vi "HH_FileToImage_2.vi"(0 "Data In":u32[](array[numeric]), 1 "Reset":bool, 2 "Image Data In":u16[][][](array[numeric]), 5 "Data Count":i32, 7 "Trigger Times":u64[](array[numeric]), 9 "Trigger":dbl[](array[numeric])) -> (3 "Image Data Out":u16[][][](array[numeric]), 6 "Total Photon Count":u64[](array[numeric]), 13 "Total Oveflow Count":u64, 14 "Num Records Total":i64)   [LabVIEW 2009]
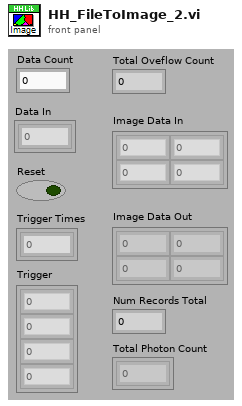
[diagram p1: front panel]
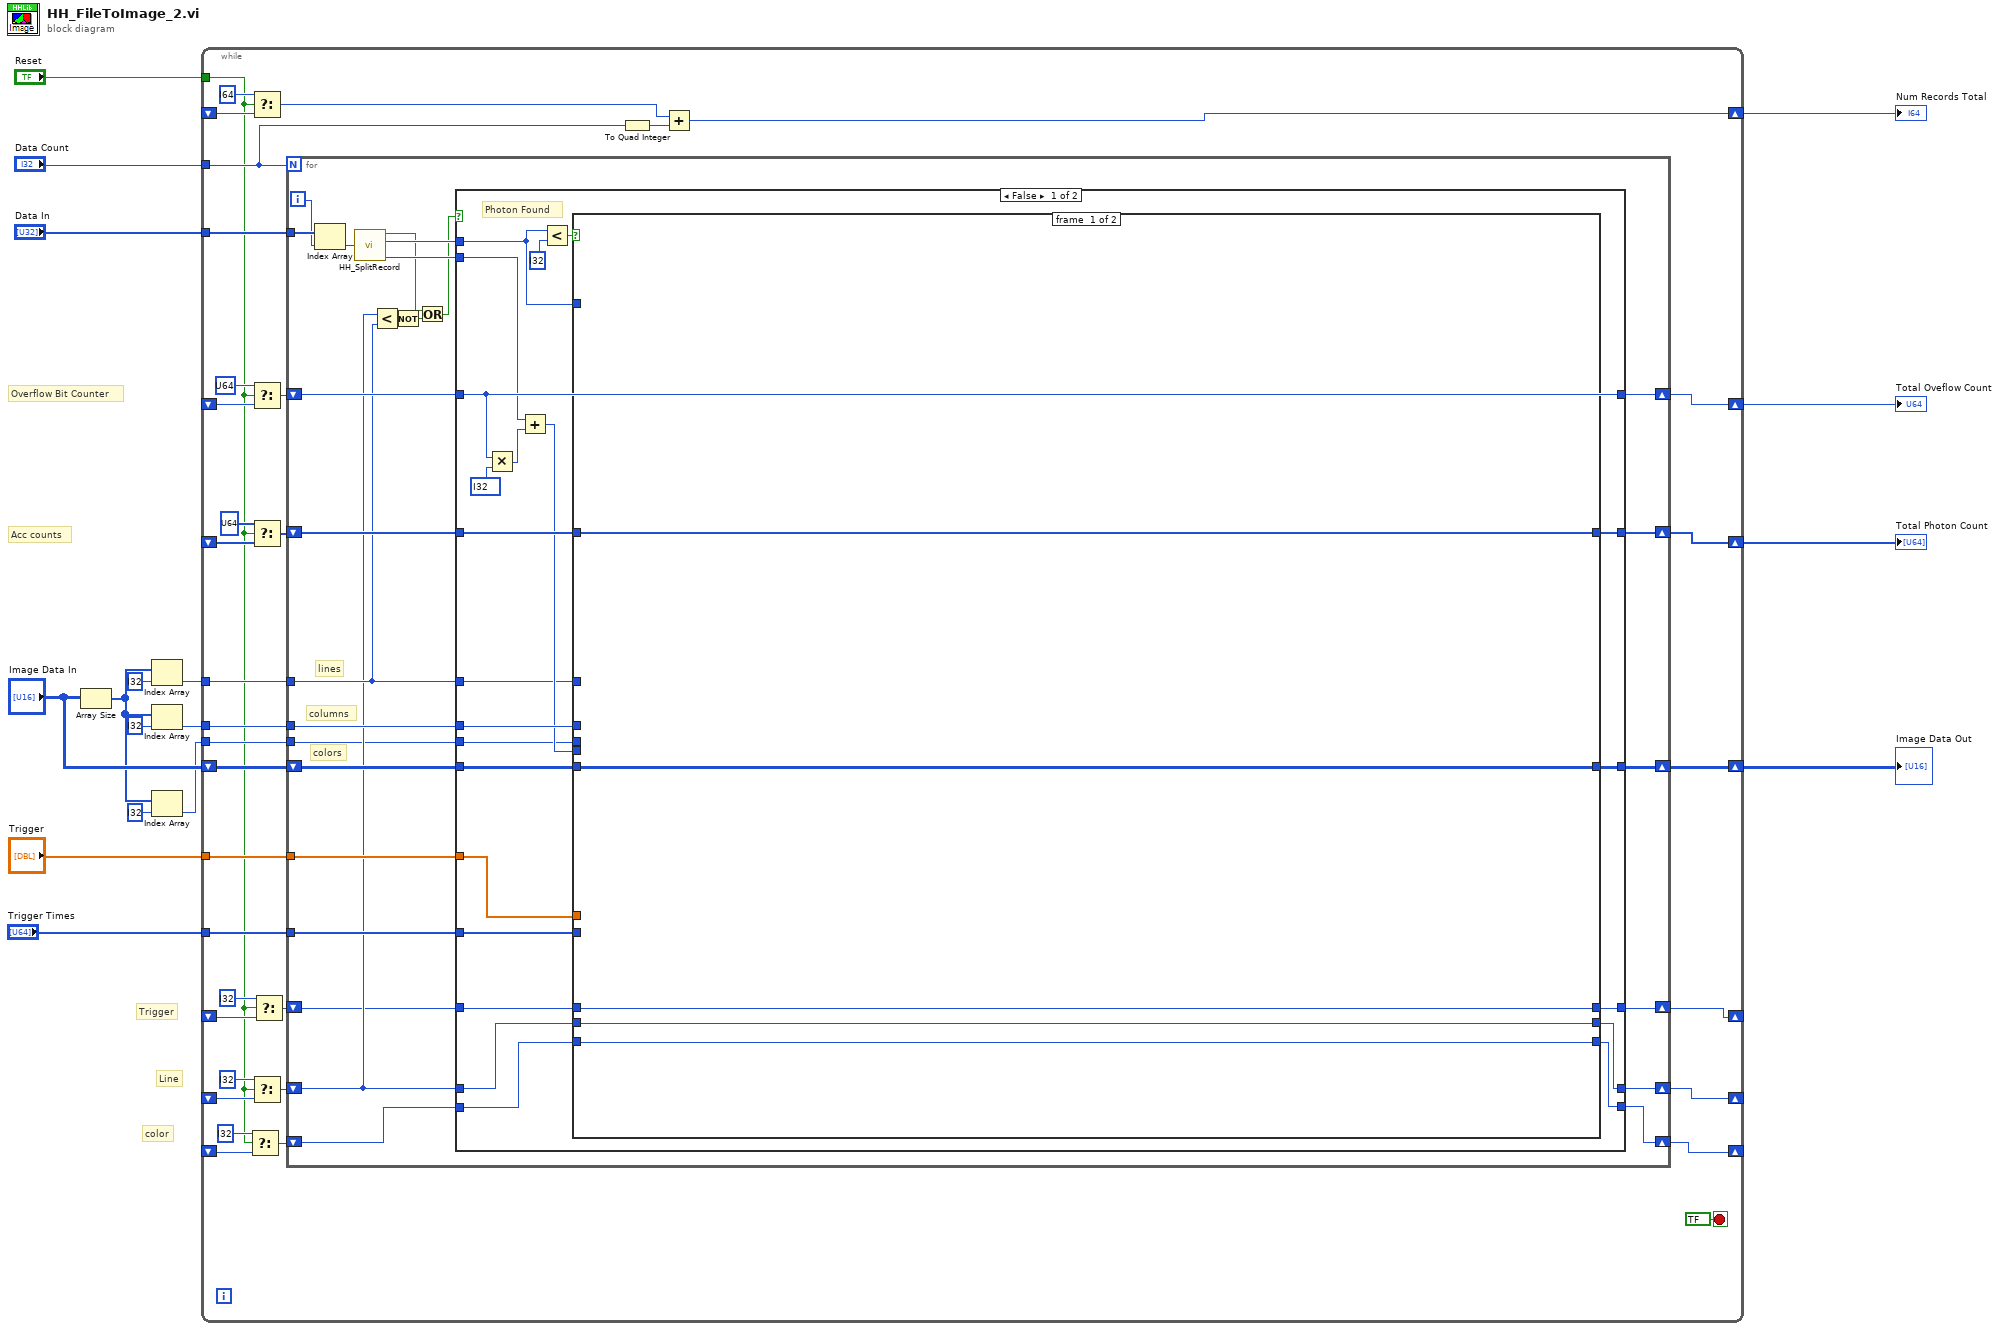
[diagram p0: block diagram]
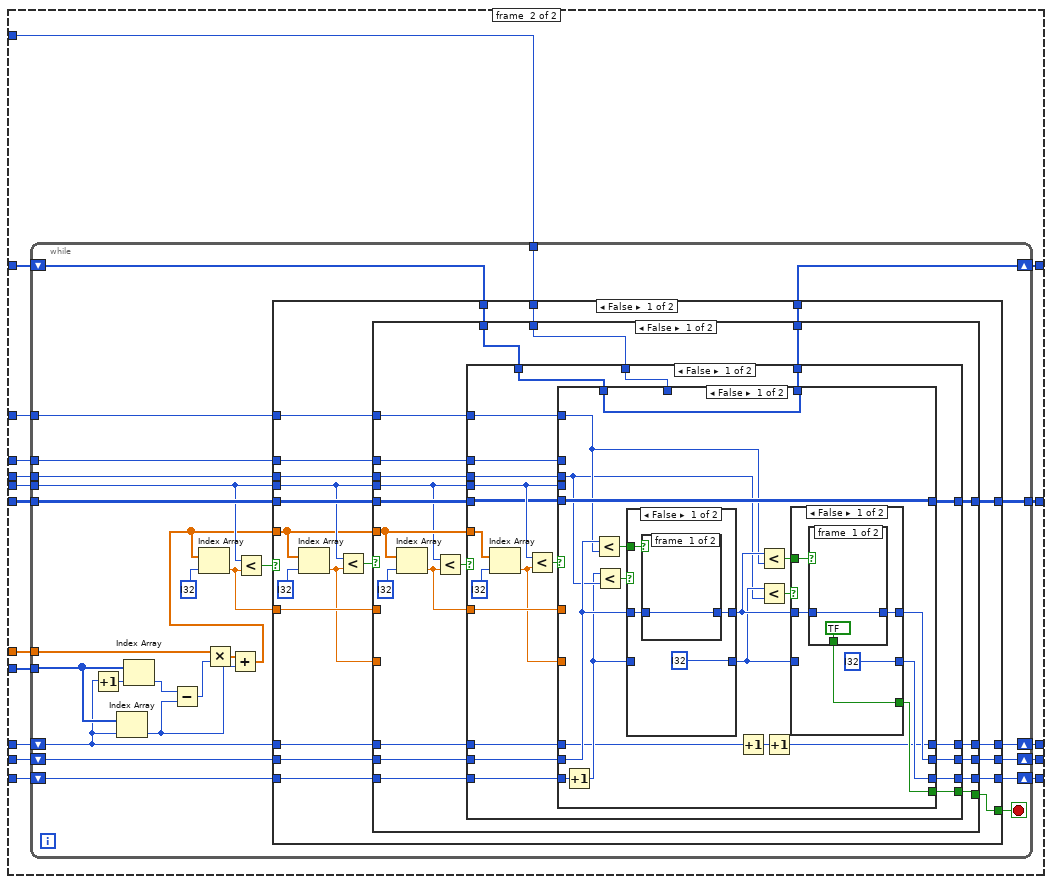
[diagram p2: hidden frame]
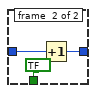
[diagram p3: hidden frame]
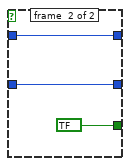
[diagram p4: hidden frame]
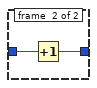
[diagram p5: hidden frame]
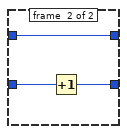
[diagram p6: hidden frame]
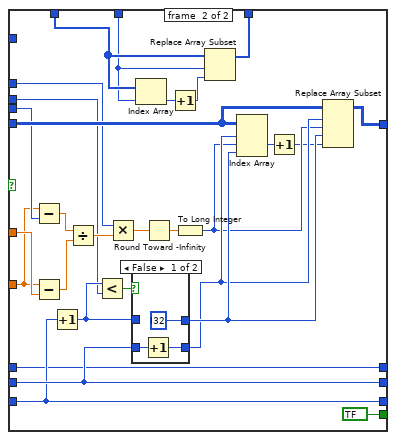
[diagram p7: hidden frame]
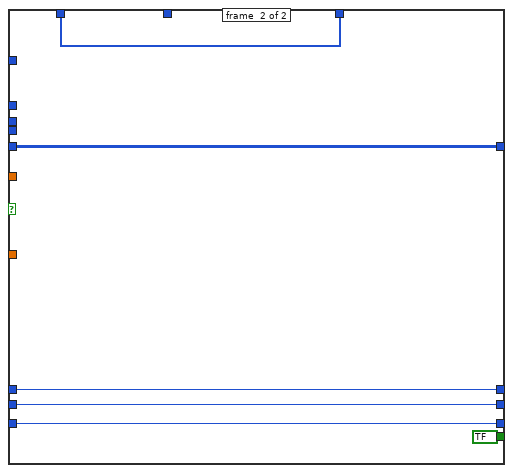
[diagram p9: hidden frame]
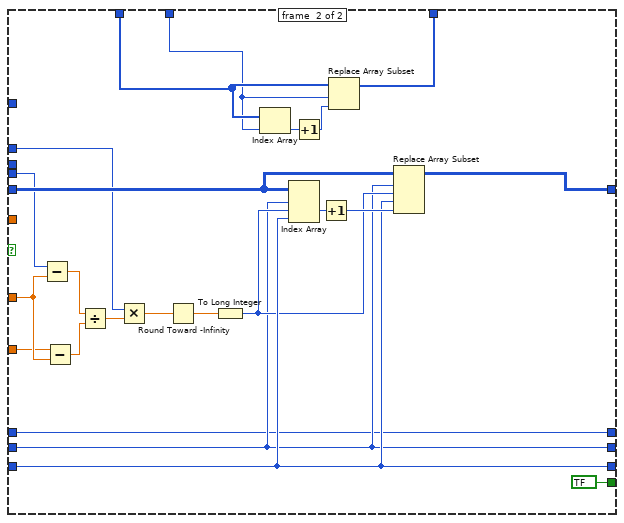
[diagram p10: hidden frame]
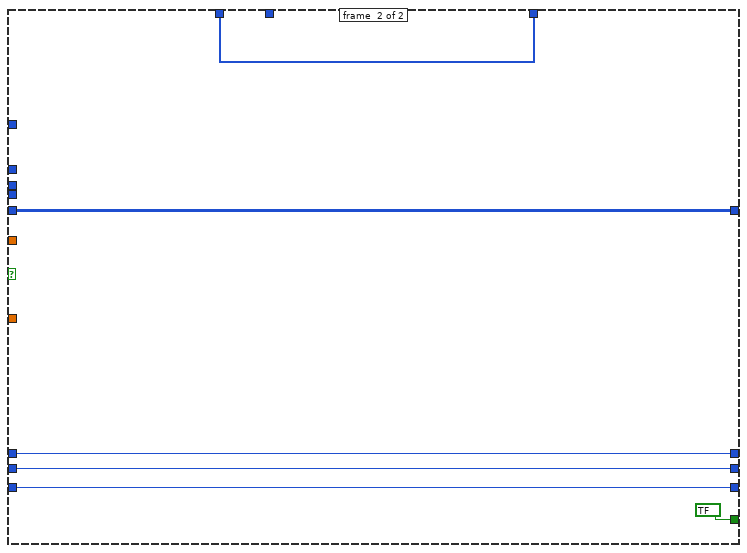
[diagram p11: hidden frame]
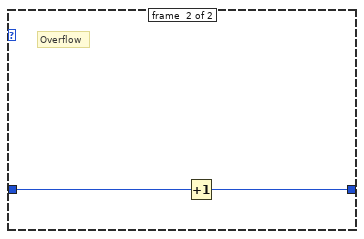
[diagram p13: hidden frame]
diagram:
  # "Trigger"
  # "color"
  # "Line"
  # "Acc counts"
  # "Overflow Bit Counter"
  n1 = Array Size(array="Image Data In") -> (size(s)=w2:i32[])
  n2 = Index Array(array=w2, index=i32 ?) -> (element=w7:i32)
  n3 = Index Array(array=w2, index=i32 ?) -> (element=w8:i32)
  n4 = Index Array(array=w2, index=i32 ?) -> (element=w1:i32)
  n5 = while {
    tunnel: "Data In" -> [w53]
    tunnel: "Reset" -> [w20]
    shift-right: [w49] -> w14
    shift-left: _ -> [w48]
    shift-right: [w45] -> _
    shift-left: _ -> [w33]
    tunnel: "Data Count" -> [w36]
    shift-right: [w41] -> w15
    shift-left: _ -> [w43]
    shift-right: [w38] -> w13
    shift-left: _ -> [w37]
    shift-right: [w34] -> w6
    shift-left: "Image Data In" -> [w32]
    tunnel: "Trigger Times" -> [w30]
    tunnel: w8 -> [w31]
    tunnel: w7 -> [w28]
    tunnel: "Trigger" -> [w29]
    shift-right: [w24] -> _
    shift-left: _ -> [w26]
    tunnel: w1 -> [w23]
    shift-right: [w19] -> _
    shift-left: _ -> [w21]
    stop <- bool ? stop-if-true
    n6 = Select(t=i32 ?, s=w20, f=w26) -> (s? t:f=w25:i32)
    n7 = Select(t=i64 ? ("Data Count 2"), s=w20, f=w43) -> (s? t:f=w42:i64)
    n8 = Select(t=u64 ?, s=w20, f=w48) -> (s? t:f=w50:u64)
    n9 = Select(t=u64[] ? ("initialized array"), s=w20, f=w37) -> (s? t:f=w39:u64[])
    n10 = Select(t=i32 ?, s=w20, f=w33) -> (s? t:f=w46:i32)
    n11 = Select(t=i32 ?, s=w20, f=w21) -> (s? t:f=w18:i32)
    n12 = for {
      N: w36 -> [_]
      tunnel: w53 -> [w77]
      shift-right: [w78] -> w49
      shift-left: w50 -> [w79]
      shift-right: [w69] -> w45
      shift-left: w46 -> [w63]
      shift-right: [w74] -> w38
      shift-left: w39 -> [w75]
      shift-right: [w70] -> w34
      shift-left: w32 -> [w71]
      tunnel: w31 -> [w65]
      tunnel: w30 -> [w66]
      tunnel: w29 -> [w67]
      tunnel: w28 -> [w64]
      shift-right: [w57] -> w24
      shift-left: w25 -> [w58]
      tunnel: w23 -> [w56]
      shift-right: [w55] -> w19
      shift-left: w18 -> [w54]
      i -> [w76]
      # "colors"
      # "lines"
      # "columns"
      n13 = Index Array(array=w77, index=w76) -> (element=w73:u32)
      n14 = call "HH_SplitRecord.vi"("Record in"=w73) -> ("Special"=w61:bool, "channel"=w72:i32, "nsync"=w68:u16)  [unwired: 1 out]
      n15 = Less?(x=w63, y=w64) -> (x < y?=w62:bool)
      n16 = Not(x=w62) -> (.not. x?=w59:bool)
      n17 = Or(x=w61, y=w59) -> (x .or. y?=w60:bool)
      n18 = case shown="False" w60 {
        tunnel: w72 -> [w94 w328]
        tunnel: w79 -> [w97 w327]
        tunnel: [w97 w326] -> w78
        tunnel: w68 -> [w92 _]
        tunnel: w75 -> [w100 w329]
        tunnel: [w99 w329] -> w74
        tunnel: w63 -> [w86 w331]
        tunnel: w71 -> [w98 w330]
        tunnel: [w93 w330] -> w70
        tunnel: [w90 w331] -> w69
        tunnel: w67 -> [w89 _]
        tunnel: w66 -> [w88 _]
        tunnel: w65 -> [w91 _]
        tunnel: w64 -> [w85 _]
        tunnel: w58 -> [w84 w325]
        tunnel: [w83 w325] -> w57
        tunnel: w56 -> [w82 _]
        tunnel: w54 -> [w81 w324]
        tunnel: [w80 w324] -> w55
        frame #0 {
          # "Photon Found"
          n19 = Multiply(x=w97, y=i32 ?) -> (x*y=w95:u64)
          n20 = Add(x=w92, y=w95) -> (x+y=w87:u64)
          n21 = Less?(x=w94, y=i32 ?) -> (x < y?=w102:bool)
          n22 = case shown="True" w102 {
            tunnel: w94 -> [_ w113]
            tunnel: w100 -> [w106 w115]
            tunnel: [w106 w114] -> w99
            tunnel: w98 -> [w107 w124]
            tunnel: [w107 w123] -> w93
            tunnel: w87 -> [_ w122]
            tunnel: w86 -> [w105 w121]
            tunnel: w91 -> [_ w120]
            tunnel: [w105 w119] -> w90
            tunnel: w85 -> [_ w118]
            tunnel: w89 -> [_ w117]
            tunnel: w88 -> [_ w116]
            tunnel: w84 -> [w104 w112]
            tunnel: [w104 w111] -> w83
            tunnel: w82 -> [_ w110]
            tunnel: w81 -> [w103 w109]
            tunnel: [w103 w108] -> w80
            frame #0 {
            }
            frame #1 {
              n23 = while {
                tunnel: w124 -> [w151]
                tunnel: [w150] -> w123
                tunnel: w122 -> [w147]
                tunnel: w120 -> [w146]
                shift-right: [w144] -> w119
                shift-left: w121 -> [w128]
                tunnel: w118 -> [w142]
                tunnel: w117 -> [w135]
                tunnel: w116 -> [w134]
                tunnel: w113 -> [w131]
                shift-right: [w132] -> w114
                shift-left: w115 -> [w133]
                shift-right: [w130] -> w111
                shift-left: w112 -> [w129]
                tunnel: w110 -> [w127]
                shift-right: [w125] -> w108
                shift-left: w109 -> [w126]
                stop <- w148 stop-if-true
                n24 = Increment(x=w126) -> (x+1=w141:i32)
                n25 = Index Array(array=w134, index=w126) -> (element=w138:u64)
                n26 = Index Array(array=w134, index=w141) -> (element=w140:u64)
                n27 = Subtract(x=w140, y=w138) -> (x-y=w139:u64)
                n28 = Multiply(x=w135, y=w139) -> (x*y=w137:dbl[])
                n29 = Add(x=w137, y=w138) -> (x+y=w136:dbl[])
                n30 = Index Array(array=w136, index=i32 ?) -> (element=w145:dbl)
                n31 = Less?(x=w147, y=w145) -> (x < y?=w149:bool)
                n32 = case shown="False" w149 {
                  tunnel: w151 -> [w170 w323]
                  tunnel: [w169 w323] -> w150
                  tunnel: w136 -> [w162 _]
                  tunnel: [w161 bool ?] -> w148
                  tunnel: w147 -> [w164 _]
                  tunnel: w128 -> [w168 w321]
                  tunnel: w146 -> [w167 _]
                  tunnel: w145 -> [w166 _]
                  tunnel: [w163 w321] -> w144
                  tunnel: w142 -> [w160 _]
                  tunnel: w133 -> [w159 w320]
                  tunnel: [w158 w320] -> w132
                  tunnel: w131 -> [w157 _]
                  tunnel: w129 -> [w156 w319]
                  tunnel: [w155 w319] -> w130
                  tunnel: w127 -> [w154 _]
                  tunnel: [w153 w318] -> w125
                  tunnel: w126 -> [w152 w318]
                  frame #0 {
                    n33 = Index Array(array=w162, index=i32 ?) -> (element=w165:dbl)
                    n34 = Less?(x=w164, y=w165) -> (x < y?=w171:bool)
                    n35 = case shown="False" w171 {
                      tunnel: w170 -> [w187 w315]
                      tunnel: [w186 w314] -> w169
                      tunnel: w168 -> [w190 w296]
                      tunnel: w167 -> [w182 w300]
                      tunnel: w166 -> [_ w305]
                      tunnel: w165 -> [_ w304]
                      tunnel: w164 -> [w184 w306]
                      tunnel: [w189 w296] -> w163
                      tunnel: w162 -> [w185 _]
                      tunnel: [w188 bool ?] -> w161
                      tunnel: w160 -> [w181 _]
                      tunnel: w159 -> [w179 w309]
                      tunnel: [w180 w308] -> w158
                      tunnel: w157 -> [w178 w307]
                      tunnel: w156 -> [w177 w298]
                      tunnel: [w176 w298] -> w155
                      tunnel: w154 -> [w175 _]
                      tunnel: [w174 w295] -> w153
                      tunnel: w152 -> [w173 w295]
                      frame #0 {
                        n36 = Index Array(array=w185, index=i32 ?) -> (element=w183:dbl)
                        n37 = Less?(x=w184, y=w183) -> (x < y?=w191:bool)
                        n38 = case shown="False" w191 {
                          tunnel: w190 -> [w206 w294]
                          tunnel: [w205 w294] -> w189
                          tunnel: [w202 bool ?] -> w188
                          tunnel: w187 -> [w204 w292]
                          tunnel: [w203 w292] -> w186
                          tunnel: w185 -> [w212 _]
                          tunnel: w184 -> [w207 _]
                          tunnel: w183 -> [w210 _]
                          tunnel: w182 -> [w208 _]
                          tunnel: w181 -> [w201 _]
                          tunnel: [w198 w291] -> w180
                          tunnel: w179 -> [w200 w291]
                          tunnel: w178 -> [w199 _]
                          tunnel: w177 -> [w197 w290]
                          tunnel: [w196 w290] -> w176
                          tunnel: w175 -> [w195 _]
                          tunnel: [w194 w289] -> w174
                          tunnel: w173 -> [w193 w289]
                          frame #0 {
                            n39 = Index Array(array=w212, index=i32 ?) -> (element=w209:dbl)
                            n40 = Less?(x=w207, y=w209) -> (x < y?=w211:bool)
                            n41 = case shown="False" w211 {
                              tunnel: w210 -> [_ w271]
                              tunnel: w209 -> [_ w267]
                              tunnel: w208 -> [_ w272]
                              tunnel: w207 -> [_ w268]
                              tunnel: w206 -> [w228 w266]
                              tunnel: [w224 w266] -> w205
                              tunnel: w204 -> [w231 w282]
                              tunnel: [w231 w281] -> w203
                              tunnel: [w223 bool ?] -> w202
                              tunnel: w201 -> [w220 _]
                              tunnel: w200 -> [w230 w277]
                              tunnel: w199 -> [_ w276]
                              tunnel: [w230 w275] -> w198
                              tunnel: w197 -> [w227 w265]
                              tunnel: [w225 w265] -> w196
                              tunnel: w195 -> [w218 w263]
                              tunnel: [w214 w256] -> w194
                              tunnel: w193 -> [w216 w256]
                              frame #0 {
                                n42 = Increment(x=w227) -> (x+1=w217:i32)
                                n43 = Less?(x=w228, y=w220) -> (x < y?=w232:bool)
                                n44 = Less?(x=w217, y=w218) -> (x < y?=w229:bool)
                                n45 = case shown="False" w229 {
                                tunnel: w232 -> [w249 _]
                                tunnel: w228 -> [w248 w255]
                                tunnel: [w247 w255] -> w221
                                tunnel: w217 -> [_ w254]
                                tunnel: [i32 ? w253] -> w219
                                frame #0 {
                                n46 = case shown="True" w249 {
                                tunnel: w248 -> [w250 w252]
                                tunnel: [w250 w251] -> w247
                                frame #0 {
                                }
                                frame #1 {
                                n47 = Increment(x=w252) -> (x+1=w251:i32)
                                }
                                }
                                }
                                frame #1 {
                                n48 = Increment(x=w254) -> (x+1=w253:i32)
                                }
                                }
                                n49 = Increment(x=w216) -> (x+1=w215:i32)
                                n50 = Less?(x=w221, y=w220) -> (x < y?=w222:bool)
                                n51 = Less?(x=w219, y=w218) -> (x < y?=w226:bool)
                                n52 = Increment(x=w215) -> (x+1=w214:i32)
                                n53 = case shown="False" w226 {
                                tunnel: w219 -> [_ w243]
                                tunnel: [i32 ? w243] -> w225
                                tunnel: w221 -> [w236 w245]
                                tunnel: [w235 w245] -> w224
                                tunnel: [w233 bool ?] -> w223
                                tunnel: w222 -> [w234 _]
                                frame #0 {
                                n54 = case shown="True" w234 {
                                tunnel: w236 -> [w239 w240]
                                tunnel: [w239 w242] -> w235
                                tunnel: [bool ? bool ?] -> w233
                                frame #0 {
                                }
                                frame #1 {
                                n55 = Increment(x=w240) -> (x+1=w242:i32)
                                }
                                }
                                }
                                frame #1 {
                                }
                                }
                              }
                              frame #1 {
                                n56 = Subtract(x=w267, y=w268) -> (x-y=w273:dbl)
                                n57 = Subtract(x=w267, y=w271) -> (x-y=w270:dbl)
                                n58 = Increment(x=w265) -> (x+1=w264:i32)
                                n59 = Divide(x=w273, y=w270) -> (x/y=w269:dbl)
                                n60 = Less?(x=w264, y=w263) -> (x < y?=w262:bool)
                                n61 = Multiply(x=w272, y=w269) -> (x*y=w274:dbl)
                                n62 = case shown="False" w262 {
                                tunnel: w266 -> [w286 w288]
                                tunnel: [w285 w288] -> w260
                                tunnel: w264 -> [_ w287]
                                tunnel: [i32 ? w287] -> w261
                                frame #0 {
                                n63 = Increment(x=w286) -> (x+1=w285:i32)
                                }
                                frame #1 {
                                }
                                }
                                n64 = Index Array(array=w277, index=w276) -> (element=w279:u64)
                                n65 = Round Toward -Infinity(1:w274) -> (0:w283:dbl)
                                n66 = Increment(x=w279) -> (x+1=w278:u64)
                                n67 = To Long Integer(number=w283) -> (32bit integer=w259:i32)
                                n68 = Replace Array Subset(array=w277, new element=w278, index=w276) -> (w275:u64[])
                                n69 = Index Array(array=w282, index (dim 0)=w260, index (dim 1)=w259, index (dim 2)=w261) -> (element=w258:u16)
                                n70 = Increment(x=w258) -> (x+1=w257:u16)
                                n71 = Replace Array Subset(array=w282, new element=w257, index (dim 0)=w260, index (dim 1)=w259, index (dim 2)=w261) -> (w281:u16[][][])
                              }
                            }
                          }
                          frame #1 {
                          }
                        }
                      }
                      frame #1 {
                        n72 = Subtract(x=w306, y=w305) -> (x-y=w302:dbl)
                        n73 = Subtract(x=w304, y=w305) -> (x-y=w303:dbl)
                        n74 = Divide(x=w302, y=w303) -> (x/y=w301:dbl)
                        n75 = Multiply(x=w300, y=w301) -> (x*y=w299:dbl)
                        n76 = Round Toward -Infinity(1:w299) -> (0:w313:dbl)
                        n77 = To Long Integer(number=w313) -> (32bit integer=w297:i32)
                        n78 = Index Array(array=w309, index=w307) -> (element=w311:u64)
                        n79 = Index Array(array=w315, index (dim 0)=w296, index (dim 1)=w297, index (dim 2)=w298) -> (element=w317:u16)
                        n80 = Increment(x=w311) -> (x+1=w310:u64)
                        n81 = Increment(x=w317) -> (x+1=w316:u16)
                        n82 = Replace Array Subset(array=w309, new element=w310, index=w307) -> (w308:u64[])
                        n83 = Replace Array Subset(array=w315, new element=w316, index (dim 0)=w296, index (dim 1)=w297, index (dim 2)=w298) -> (w314:u16[][][])
                      }
                    }
                  }
                  frame #1 {
                  }
                }
              }
            }
          }
        }
        frame #1 {
          # "Special Event"
          n84 = case shown="63" w328 {
            tunnel: w327 -> [w332 w334]
            tunnel: [w332 w333] -> w326
            frame #0 {
            }
            frame #1 {
              # "Overflow"
              n85 = Increment(x=w334) -> (x+1=w333:u64)
            }
          }
        }
      }
    }
    n86 = To Quad Integer(1:w36) -> (0:w35:i64)
    n87 = Add(x=w42, y=w35) -> (x+y=w41:i64)
  }
  "Num Records Total" <- w15
  "Total Oveflow Count" <- w14
  "Total Photon Count" <- w13
  "Image Data Out" <- w6
